vi "Find_calibration_file.vi"(1 "Inst type":T1=enum."Pressure Transducer", 2 "Ch No":i16, 3 "Use Latest Calib":bool, 4 "filename":path) -> (0 "filename out":path)   [LabVIEW 2010]
uses:
  Controls/Inst_type.ctl
  Controls/App_Global.ctl
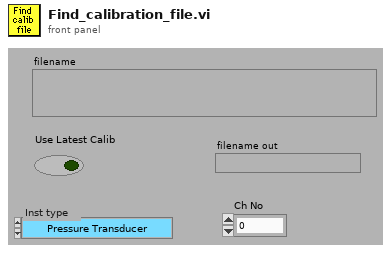
[diagram p1: front panel]
types:
  T1 = typedef "Inst_type.ctl" = enum16{"Propeller anemometer", "Raw voltage", "Pressure Transducer", "Pitot-static tube", "Preston tube", "Hot wire", "Cross wire 1", "Cross wire 2", "Generic Linear", "Generic Polynomial", "Generic BackPoly", "Fast FID", "Thermocouple", "Cold wire", "Pulsed Wire", "LDA Vel", "LDA Tran time", "LDA Arr time"}
  T2 = typedef "App_Global.ctl" = enum16{"Read Global", "Write to Global", "Initialise Array"}
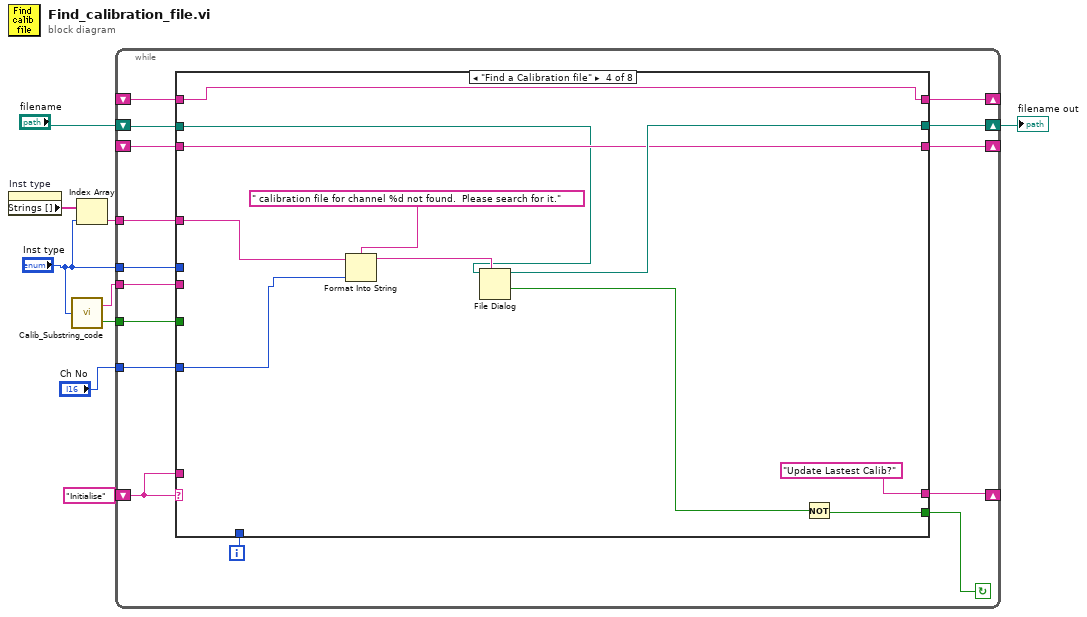
[diagram p0: block diagram]
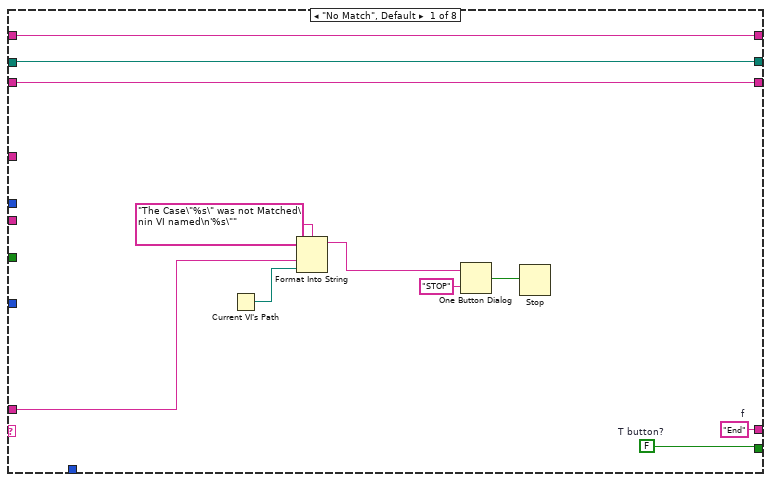
[diagram p2: hidden frame]
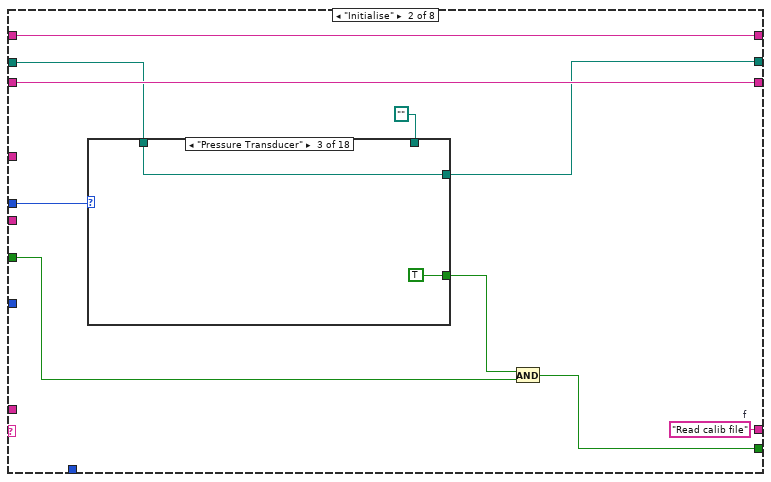
[diagram p3: hidden frame]
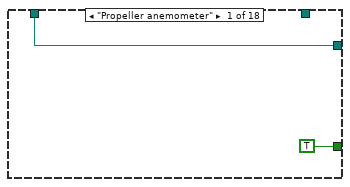
[diagram p4: hidden frame]
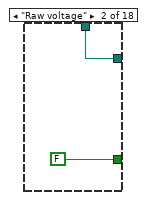
[diagram p5: hidden frame]
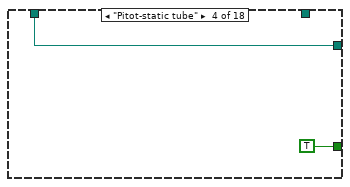
[diagram p6: hidden frame]
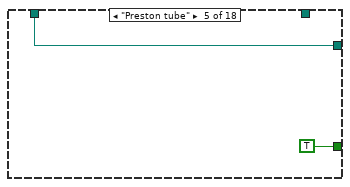
[diagram p7: hidden frame]
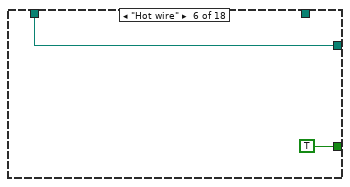
[diagram p8: hidden frame]
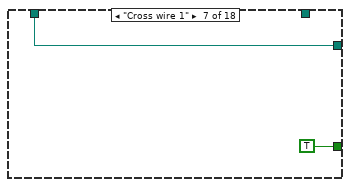
[diagram p9: hidden frame]
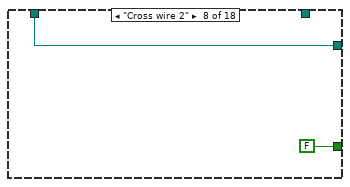
[diagram p10: hidden frame]
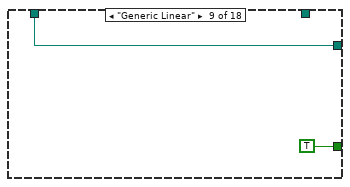
[diagram p11: hidden frame]
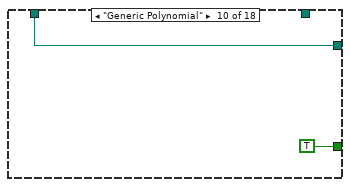
[diagram p12: hidden frame]
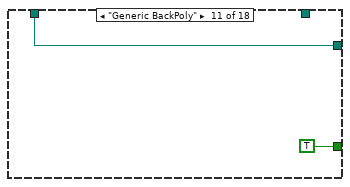
[diagram p13: hidden frame]
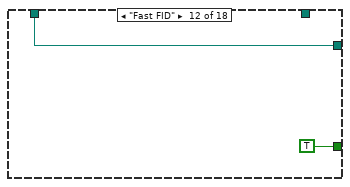
[diagram p14: hidden frame]
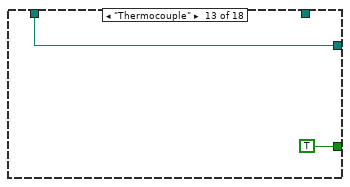
[diagram p15: hidden frame]
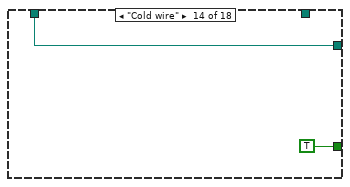
[diagram p16: hidden frame]
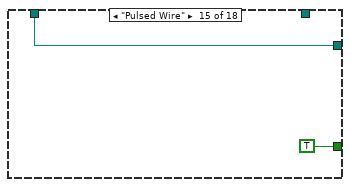
[diagram p17: hidden frame]
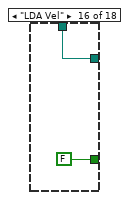
[diagram p18: hidden frame]
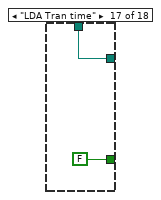
[diagram p19: hidden frame]
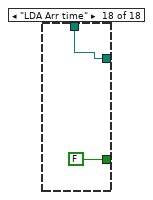
[diagram p20: hidden frame]
diagram:
  n1 = property on="Inst type" class="Enum (strict)"() -> ("Strings []"=w6:string[])  [unwired: 2 in, 2 out]
  n2 = call "Calib_Substring_code.vi"("Inst type"="Inst type") -> ("Substring Type"=w3:string, "Read file"=w2:bool)
  n3 = Index Array(array=w6, index="Inst type") -> (element=w5:string)
  n4 = while {
    shift-left: "filename" -> [w24]
    shift-right: [w23] -> w8
    shift-left: "Initialise" -> [w17]
    shift-right: [w22] -> _
    shift-right: [w19] -> _
    shift-left: _ -> [w18]
    tunnel: "Inst type" -> [w16]
    tunnel: w5 -> [w15]
    shift-right: [w13] -> _
    shift-left: _ -> [w14]
    tunnel: w3 -> [w12]
    tunnel: w2 -> [w11]
    tunnel: "Ch No" -> [w10]
    i -> [w20]
    stop <- w21 continue-if-true
    n5 = case shown="\"Find a Calibration file\"" w17 {
      tunnel: w24 -> [w34 w40 w89 w90 w102 w124 w157 w186]
      tunnel: [w34 w41 w89 w100 w102 w124 w157 w186] -> w23
      tunnel: [w33 w42 w85 "Update Lastest Calib?" w107 w136 "Find a Calibration file" "Read calib file" ("f")] -> w22
      tunnel: [w32 w36 TRUE w96 w110 w137 w172 w184] -> w21
      tunnel: w20 -> [_ _ _ _ _ _ _ _]
      tunnel: [w35 w45 w84 w99 w105 w134 w159 w188] -> w19
      tunnel: w18 -> [w35 w45 _ w99 w105 w134 w159 w188]
      tunnel: w17 -> [w26 _ _ _ _ _ _ _]
      tunnel: w16 -> [_ w43 _ _ _ w135 _ _]
      tunnel: w15 -> [_ _ _ w94 w108 _ _ _]
      tunnel: w14 -> [w25 w44 w82 w95 _ w133 w160 w187]
      tunnel: [w25 w44 w82 w95 w106 w133 w160 w187] -> w13
      tunnel: w12 -> [_ _ _ _ w104 _ _ _]
      tunnel: w11 -> [_ w37 _ _ _ _ _ _]
      tunnel: w10 -> [_ _ _ w91 _ _ _ w183]
      frame "No Match", Default {
        w32 = FALSE  # T button?
        w33 = "End"  # f
        n6 = Current VI's Path() -> (path=w27:path)
        n7 = Format Into String(format string="The Case\"%s\" was not Matched\nin VI named\n'%s\"" ("Format String"), w26, w27) -> (resulting string=w30:string)  [unwired: 2 in, 1 out]
        n8 = One Button Dialog(message=w30, button name ("OK")="STOP") -> (true=w28:bool)
        n9 = Stop(stop? (T)=w28) -> ()
      }
      frame "Initialise" {
        w42 = "Read calib file"  # f
        n10 = case shown="\"Pressure Transducer\"" w43 {
          tunnel: [TRUE FALSE TRUE TRUE TRUE TRUE TRUE FALSE TRUE TRUE TRUE TRUE TRUE TRUE TRUE FALSE FALSE FALSE] -> w38
          tunnel: [w46 w48 w50 w52 w54 w56 w58 w60 w62 w64 w66 w68 w70 w72 w74 w76 w78 w80] -> w41
          tunnel: w40 -> [w46 _ w50 w52 w54 w56 w58 w60 w62 w64 w66 w68 w70 w72 w74 _ _ _]
          tunnel: path "" -> [_ w48 _ _ _ _ _ _ _ _ _ _ _ _ _ w76 w78 w80]
          frame "Propeller anemometer" {
          }
          frame "Raw voltage" {
          }
          frame "Pressure Transducer" {
          }
          frame "Pitot-static tube" {
          }
          frame "Preston tube" {
          }
          frame "Hot wire" {
          }
          frame "Cross wire 1" {
          }
          frame "Cross wire 2" {
          }
          frame "Generic Linear" {
          }
          frame "Generic Polynomial" {
          }
          frame "Generic BackPoly" {
          }
          frame "Fast FID" {
          }
          frame "Thermocouple" {
          }
          frame "Cold wire" {
          }
          frame "Pulsed Wire" {
          }
          frame "LDA Vel" {
          }
          frame "LDA Tran time" {
          }
          frame "LDA Arr time" {
          }
        }
        n11 = And(x=w38, y=w37) -> (x .and. y?=w36:bool)
      }
      frame "Read calib file" {
        w83 = "Check for calib substring"  # f
        n12 = call "Read_File_Simple.vi"("Filename"=w89) -> ("Error?"=w87:bool, "string"=w84:string)  [unwired: 2 in, 6 out]
        n13 = Select(t="Find a Calibration file", s=w87, f=w83) -> (s? t:f=w85:string)
      }
      frame "Find a Calibration file" {
        n14 = Format Into String(format string=" calibration file for channel %d not found.  Please search for it.", initial string=w94, w91) -> (resulting string=w92:string)  [unwired: 1 in, 1 out]
        n15 = File Dialog(7:w92, 11:w90) -> (1:w97:bool, 3:w100:path)  [unwired: 1 in, 6 out]
        n16 = Not(x=w97) -> (.not. x?=w96:bool)
      }
      frame "Check for calib substring" {
        w112 = FALSE  # Show Dialog?
        n17 = Concatenate Strings(w104, "calib label") -> (w109:string)
        n18 = Format Into String(format string="Calibration File   %s", w102) -> (resulting string=w101:string)  [unwired: 2 in, 1 out]
        n19 = call "Get_string_subset.vi"("String Name"=w101, "Show Dialog?"=w112, "String to split"=w105, "File Label"=w109) -> ("Status"=w111:enum16{"Char in string", "Char not in string"}, "Output string"=w106:string)
        n20 = case shown="\"Char in string\"" w111 {
          tunnel: [TRUE w121] -> w110
          tunnel: w102 -> [_ w117]
          tunnel: w108 -> [_ w120]
          tunnel: ["Was there sufficient calibration points?" "Find a Calibration file"] -> w107
          frame "Char in string" {
          }
          frame "Char not in string" {
            w118 = "The calibration file\n\"%s\"\nis not the appropriate file for a %s"  # format string
            w122 = "Find another file"  # T button name ("OK")
            n21 = Strip Path(path=w117) -> (name=w116:string)  [unwired: 1 out]
            n22 = Format Into String(format string=w118, w116, w120) -> (resulting string=w123:string)  [unwired: 2 in, 1 out]
            n23 = Two Button Dialog(message=w123, 2:w122) -> (T button?=w121:bool)  [unwired: 1 out]
          }
        }
      }
      frame "Was there sufficient calibration points?" {
        n24 = Format Into String(format string="Calibration File   %s", w124) -> (resulting string=w125:string)  [unwired: 2 in, 1 out]
        n25 = call "2D_array_from_string.vi"("String Name"=w125, "Input string"=w133, "Array title"="Calib points label") -> ("2D data array"=w132:dbl[][])  [unwired: 1 in]
        n26 = for {
          tunnel: w132 -> [w143] mode=indexing
          tunnel: [w139] -> w128 mode=indexing
          n27 = Index Array(array=w143, index=5) -> (element=w141:dbl)
          n28 = Not A Number/Path/Refnum?(number/path/refnum=w141) -> (NaN/Path/Refnum?=w140:bool)
          n29 = Not(x=w140) -> (.not. x?=w139:bool)
        }
        n30 = Boolean To (0,1)(Boolean=w128) -> (0, 1=w131:i16[])
        n31 = Add Array Elements(numeric array=w131) -> (sum=w129:i16)
        n32 = Greater?(x=w129, y=i16 1) -> (0:w127:bool)
        n33 = case shown="True" w127 {
          tunnel: [w148 w152] -> w137
          tunnel: w124 -> [w145 _]
          tunnel: ["Find a Calibration file" "Are XW psi 1 and 2 valid"] -> w136
          tunnel: w135 -> [_ w153]
          frame False {
            w146 = "The calibration file\n\"%s\"\nhas less than two calibration points."  # format string
            w149 = "Find another file"  # T button name ("OK")
            n34 = Strip Path(path=w145) -> (name=w144:string)  [unwired: 1 out]
            n35 = Format Into String(format string=w146, w144) -> (resulting string=w150:string)  [unwired: 2 in, 1 out]
            n36 = Two Button Dialog(message=w150, 2:w149) -> (T button?=w148:bool)  [unwired: 1 out]
          }
          frame True {
            n37 = case shown="\"Propeller anemometer\", Default" w153 {
              tunnel: [FALSE TRUE] -> w152
              frame "Propeller anemometer", Default {
              }
              frame "Cross wire 1" {
              }
            }
          }
        }
      }
      frame "Are XW psi 1 and 2 valid" {
        w165 = FALSE  # Show Dialog?
        n38 = Build Array("C0", "C1", "C2") -> (w167:string[])
        n39 = Format Into String(format string="Calibration File   %s", w157) -> (resulting string=w156:string)  [unwired: 2 in, 1 out]
        n40 = call "Get_string_subset.vi"("String Name"=w156, "Show Dialog?"=w165, "String to split"=w159, "File Label"="Auxiliary constants") -> ("Output string"=w166:string)  [unwired: 1 out]
        n41 = for {
          tunnel: w167 -> [w175] mode=indexing
          tunnel: [w174] -> w164 mode=indexing
          tunnel: w166 -> [w173]
          n42 = call "Get_value_from_string.vi"("Input string"=w173, "Variable name"=w175) -> ("Value"=w174:dbl)  [unwired: 1 in, 1 out]
        }
        n43 = Not A Number/Path/Refnum?(number/path/refnum=w164) -> (NaN/Path/Refnum?=w163:bool[])
        n44 = Or Array Elements(Boolean array=w163) -> (logical OR=w162:bool)
        n45 = case shown="False" w162 {
          tunnel: [FALSE w180] -> w172
          tunnel: w157 -> [_ w178]
          frame False {
          }
          frame True {
            n46 = Strip Path(path=w178) -> (name=w177:string)  [unwired: 1 out]
            n47 = Format Into String(format string="The XW calibration file\n\"%s\"\ndoes not have valid angle calibration coefficients.", w177) -> (resulting string=w182:string)  [unwired: 2 in, 1 out]
            n48 = Two Button Dialog(message=w182, 2:"Find another file" ("T button name (\"OK\")")) -> (T button?=w180:bool)  [unwired: 1 out]
          }
        }
      }
      frame "Update Lastest Calib?" {
        w184 = TRUE  # T button?
        n49 = case shown="True" "Use Latest Calib" {
          tunnel: w186 -> [_ w193]
          tunnel: w183 -> [_ w190]
          frame False {
          }
          frame True {
            n50 = Build Array(w193) -> (w191:path[])
            n51 = Build Array(w190) -> (w192:i16[])
            n52 = call "Current_Calib_Filenames.vi"("Calib Filename"=w191, "Channel Numbers"=w192, "Mode"=App_Global."Write to Global") -> ()  [unwired: 3 out]
          }
        }
      }
    }
  }
  "filename out" <- w8
